vi "Percent of Full Screen.vi"(8 "error in (no error)":errorcluster) -> (0 "error out":errorcluster, 2 "Bottom":i16, 3 "Right":i16)   [LabVIEW 2014]
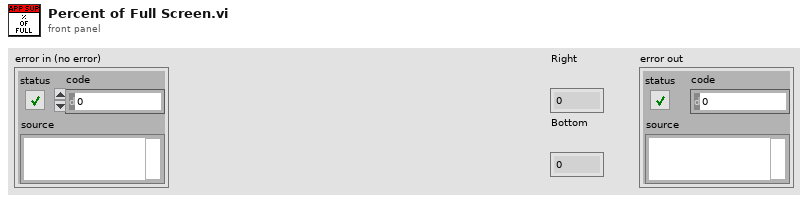
[diagram p1: front panel]
types:
  T1 = typedef "LVRectTypeDef.ctl" = cluster{"Left":i16, "Top":i16, "Right":i16, "Bottom":i16}
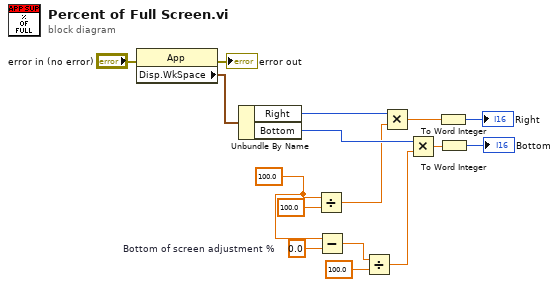
[diagram p0: block diagram]
diagram:
  w4 = 0.0  # Bottom of screen adjustment %
  w5 = 100.0 ("x")
  n1 = property class="App"(error in="error in (no error)") -> (error out=→"error out":errorcluster, "Disp.WkSpace"=w16:T1)  [unwired: 1 in, 1 out]
  n2 = Unbundle By Name(w16) -> ("Right"=w13:i16, "Bottom"=w12:i16)
  n3 = Divide(x=w5, y=100.0) -> (x/y=w11:dbl)
  n4 = Subtract(x=w5, y=w4) -> (x-y=w2:dbl)
  n5 = Divide(x=w2, y=100.0) -> (x/y=w1:dbl)
  n6 = Multiply(x=w13, y=w11) -> (x*y=w10:dbl)
  n7 = Multiply(x=w12, y=w1) -> (x*y=w9:dbl)
  n8 = To Word Integer(number=w10) -> (16bit integer=→"Right":i16)
  n9 = To Word Integer(number=w9) -> (16bit integer=→"Bottom":i16)
